vi "Configure Timebase.vi"(7 "Min Record Length (3: 1000)":u16(ring)=3 items=["100", "250", "500", "1000", "MAX"], 8 "error in (no error)":errorcluster, 9 "Start Time (0.0)":dbl, 10 "Timebase (20.0E-9)":dbl=2e-08 format="%^_3e", 11 "VISA resource name":refnum<visa-resource-name>) -> (0 "error out":errorcluster, 3 "VISA resource name out":refnum<visa-resource-name>)   [LabVIEW 2017, in "Agilent 6000 Series.lvlib"]
doc: "This VI configures the common properties of the acquisition subsystem. These properties are the time per record, minimum record length, and acquisition start time."
uses:
  <instrlib>/Agilent 6000 Series/Agilent 6000 Series.lvlib
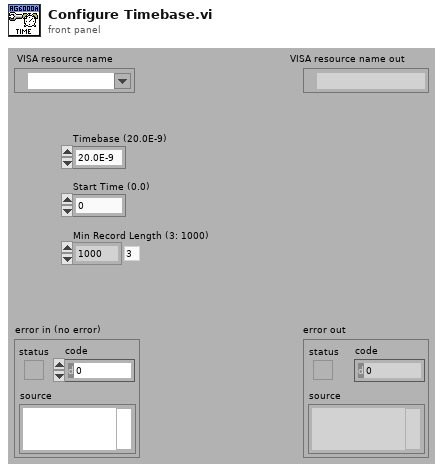
[diagram p1: front panel]
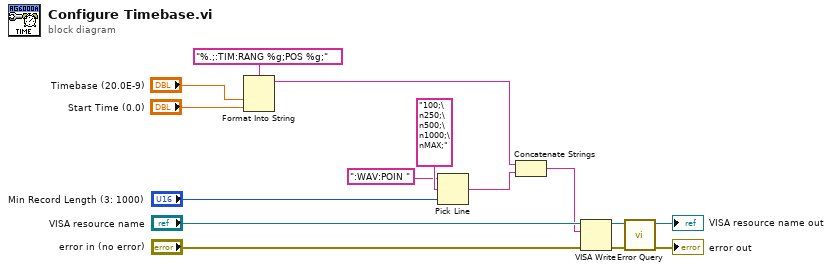
[diagram p0: block diagram]
diagram:
  n1 = Format Into String(format string="%.;:TIM:RANG %g;POS %g;", "Timebase (20.0E-9)", "Start Time (0.0)") -> (resulting string=w6:string)  [unwired: 2 in, 1 out]
  n2 = Pick Line(string ("")=":WAV:POIN ", multi-line string="100;\n250;\n500;\n1000;\nMAX;", line index="Min Record Length (3: 1000)") -> (output string=w1:string)
  n3 = Concatenate Strings(w6, w1) -> (w5:string)
  n4 = VISA Write(VISA resource name="VISA resource name", write buffer=w5, error in (no error)="error in (no error)") -> (VISA resource name out=w11:refnum<visa-resource-name>, error out=w10:errorcluster)  [unwired: 1 out]
  n5 = call <instrlib>:"Error Query.vi"("error in (no error)"=w10, "VISA resource name"=w11) -> ("error out"=→"error out":errorcluster, "VISA resource name out"=→"VISA resource name out":refnum<visa-resource-name>)  [unwired: 6 in, 2 out]
